vi "TCP Resolve IP or FQDN.vi"(1 "Machine (empty = this machine)":string) -> (0 "Resolved IP or FQDN":string)   [LabVIEW 2011]
doc: "Resolve the given machine to either an IP address or Fully Qualified Domain Name (FQDN). \n\nAcceptable input formats are: IP Address, FQDN, Machine Name, DNS Alias or Host, and Blank (this machine)."
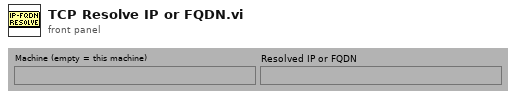
[diagram p1: front panel]
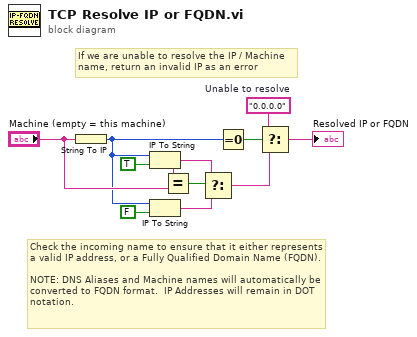
[diagram p0: block diagram]
diagram:
  w2 = "0.0.0.0"  # Unable to resolve
  # "If we are unable to resolve the IP / Machine name, return an invalid IP as an error"
  # "Check the incoming name to ensure that it either represents a valid IP address, or a Fully Qualified Domain Name (FQDN).\n\nNOTE: DNS Aliases and Machine names will automatically be converted to FQDN format.  IP Addresses will remain in DOT notation."
  n1 = String To IP(1:"Machine (empty = this machine)") -> (0:w5:u32)
  n2 = IP To String(1:TRUE ("dot notation? (F)"), 2:w5) -> (0:w7:string)
  n3 = IP To String(1:FALSE ("dot notation? (F)"), 2:w5) -> (0:w6:string)
  n4 = Equal?(x=w7, y="Machine (empty = this machine)") -> (x = y?=w8:bool)
  n5 = Select(t=w7, s=w8, f=w6) -> (s? t:f=w3:string)
  n6 = Equal To 0?(x=w5) -> (x = 0?=w4:bool)
  n7 = Select(t=w2, s=w4, f=w3) -> (s? t:f=→"Resolved IP or FQDN":string)
